vi "Reply_Package.vi"(0 "UART Reply":T1, 1 "UART_Ch":u8, 5 "Reply Data":u16) -> (4 "Reply packed":u32)   [LabVIEW 2015, in "UART_Firmware.lvlib"]
uses:
  UART_Firmware.lvlib
  UART_Response.ctl
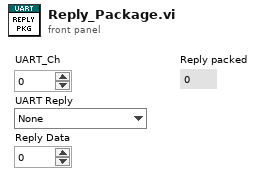
[diagram p1: front panel]
types:
  T1 = typedef "UART_Firmware.lvlib/UART_Response.ctl" = enum8{"None", "Rx", "BaudHighAck", "BaudLowAck", "CharSizeAck", "ParityAck", "StopBitsAck", "SpacingHighAck", "SpacingLowAck", "ParityError", "FrameError"}
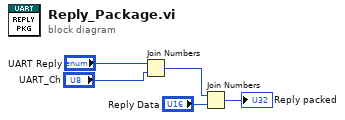
[diagram p0: block diagram]
diagram:
  n1 = Join Numbers(hi="UART Reply", lo="UART_Ch") -> ((hi.lo)=w4:u16)
  n2 = Join Numbers(hi=w4, lo="Reply Data") -> ((hi.lo)=→"Reply packed":u32)
